vi "arydh -- get all readings.vi"(7 "nanocal config":T2={"Hs"={"out"=enum."D", "shunt R (Ohm)"=100000.0, "V"={"c"=enum."A V1", "l"=enum."Lock-in set L1"}, "\"I\""={"c"=enum."A V2", "l"=enum."Lock-in set L1"}}, "ofset heater"={"out"=enum."C", "\"I\""=enum."C V2", "shunt R (Ohm)"=10000.0}, "Ts"={"out"=enum."D", "shunt R (Ohm)"=100000.0, "V"={"c"=enum."D V1", "l"=enum."Lock-in set L1"}, "\"I\""={"c"=enum."D V2", "l"=enum."Lock-in set L1"}}, "Tr"={"out"=enum."B", "shunt R (Ohm)"=100000.0, "V"={"c"=enum."E V1", "l"=enum."Lock-in set L1"}, "\"I\""={"c"=enum."E V2", "l"=enum."Lock-in set L1"}}, "Hr"={"out"=enum."E", "shunt R (Ohm)"=100000.0, "V"={"c"=enum."B V1", "l"=enum."Lock-in set L1"}, "\"I\""={"c"=enum."B V2", "l"=enum."Lock-in set L1"}}, "differential"={"c"=enum."C V1", "l"=enum."Lock-in set L2"}} {"Hr"."shunt R (Ohm)" format="%#_6p"; "Tr"."shunt R (Ohm)" format="%#_6p"; "Ts"."shunt R (Ohm)" format="%#_6p"; "ofset heater"."shunt R (Ohm)" format="%#_6p"; "Hs"."shunt R (Ohm)" format="%#_6p"}, 11 "MCL object":T7) -> (2 "engine reading":T1={"Ts -- V (V)"=100000.0+0.0i, "Hr -- V (V)"=100000.0+0.0i, "Hs -- V (V)"=100000.0+0.0i, "Tr -- V (V)"=100000.0+0.0i, "Diff -- V (V)"=100000.0+0.0i, "offset (V)"=100000.0+0.0i, "Ts -- \"I\" (V)"=100000.0+0.0i, "Hs -- \"I\" (V)"=100000.0+0.0i, "Tr -- \"I\" (V)"=100000.0+0.0i, "Hr -- \"I\" (V)"=100000.0+0.0i, "freq (Hz)"=100000.0} {"freq (Hz)" format="%#_6p"; "Hr -- \"I\" (V)" format="%#_6p"; "Tr -- \"I\" (V)" format="%#_6p"; "Hs -- \"I\" (V)" format="%#_6p"; "Ts -- \"I\" (V)" format="%#_6p"; "offset (V)" format="%#_6p"; "Diff -- V (V)" format="%#_6p"; "Tr -- V (V)" format="%#_6p"; "Hs -- V (V)" format="%#_6p"; "Hr -- V (V)" format="%#_6p"; "Ts -- V (V)" format="%#_6p"})   [LabVIEW 2018]
uses:
  nanocal/Nanocalorimetry/data/MCL.lvlibp/MCL library/MCL_DataRef.ctl
  nanocal - config.ctl
  resistoricicle.ctl
  channelicicle.ctl
  nanocal/Nanocalorimetry/data/MCL.lvlibp/SynkTek FPGA/FPGA_SharedResources/FPGASharedResources_Readings_ReadingChannelTypedef.ctl
  nanocal/Nanocalorimetry/data/MCL.lvlibp/SynkTek FPGA/FPGA_SharedResources/FPGASharedResources_Lockin_Typedef.ctl
  engine reading icicle.ctl
  nanocal/Nanocalorimetry/data/MCL.lvlibp/SynkTek FPGA/FPGA_SharedResources/FPGASharedResources_FreqCtrl_FreqGenTypedef.ctl
  nanocal/Nanocalorimetry/data/MCL.lvlibp
  nanocal/Nanocalorimetry/data/MCL.lvlibp/SynkTek FPGA/FPGA_SharedResources/FPGA_SharedResources.lvlib
panel:
  # "Ts"
  # "Tr"
  # "Hs"
  # "Hr"
  # "offset heater"
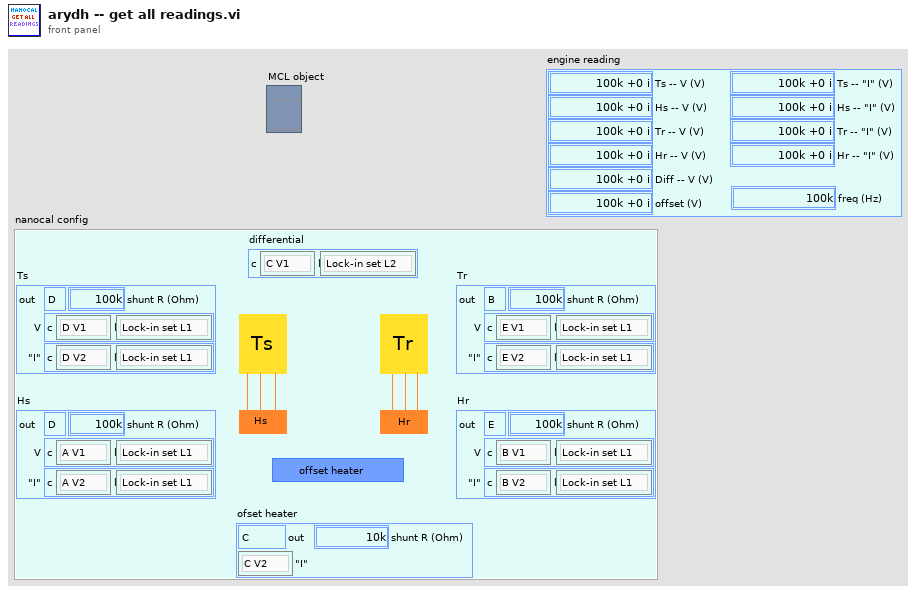
[diagram p1: front panel]
types:
  T1 = typedef "engine reading icicle.ctl" = cluster{"Ts -- V (V)":cdb, "Hr -- V (V)":cdb, "Hs -- V (V)":cdb, "Tr -- V (V)":cdb, "Diff -- V (V)":cdb, "offset (V)":cdb, "Ts -- \"I\" (V)":cdb, "Hs -- \"I\" (V)":cdb, "Tr -- \"I\" (V)":cdb, "Hr -- \"I\" (V)":cdb, "freq (Hz)":dbl}
  T2 = typedef "nanocal - config.ctl" = cluster{"Hs":T3, "ofset heater":cluster{"out":enum16{"A", "B", "C", "D", "E"}, "\"I\"":T5, "shunt R (Ohm)":dbl}, "Ts":T3, "Tr":T3, "Hr":T3, "differential":T4}
  T3 = typedef "resistoricicle.ctl" = cluster{"out":enum16{"A", "B", "C", "D", "E"}, "shunt R (Ohm)":dbl, "V":T4, "\"I\"":T4}
  T4 = typedef "channelicicle.ctl" = cluster{"c":T5, "l":T6}
  T5 = typedef "MCL.lvlibp/FPGA_SharedResources.lvlib/FPGASharedResources_Readings_ReadingChannelTypedef.ctl" = enum8{"A V1", "A V2", "B V1", "B V2", "C V1", "C V2", "D V1", "D V2", "E V1", "E V2", "A I", "B I", "C I", "D I", "E I", "Int."}
  T6 = typedef "MCL.lvlibp/FPGA_SharedResources.lvlib/FPGASharedResources_Lockin_Typedef.ctl" = enum8{"Lock-in set L1", "Lock-in set L2"}
  T7 = typedef "MCL.lvlibp/MCL_DataRef.ctl" = refnum<vi>
  T8 = typedef "MCL.lvlibp/FPGA_SharedResources.lvlib/FPGASharedResources_FreqCtrl_FreqGenTypedef.ctl" = enum8{"Frequency 1", "Frequency 2", "Frequency 3", "Frequency 4", "Frequency 5", "Frequency 6: PLL 1", "Frequency 7: PLL 2", "Frequency 8"}
  T9 = typedef "MCL.lvlibp/LIControl.lvlib/LIControl_FreqCtrl_typedef.ctl" = cluster{"Frequency (Hz)":dbl, "Ramp changes":bool, "Ramp time const. (s)":T10}
  T10 = typedef "MCL.lvlibp/LIControl.lvlib/LIControl_LockinTimeConstant_typedef.ctl" = dbl
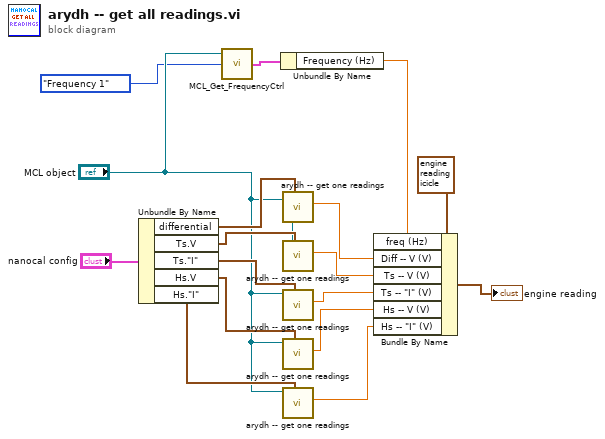
[diagram p0: block diagram]
diagram:
  n1 = Unbundle By Name("nanocal config") -> ("differential"=w15:T4, "Ts.V"=w13:T4, "Ts.\"I\""=w11:T4, "Hs.V"=w9:T4, "Hs.\"I\""=w8:T4)
  n2 = call "MCL_Get_FrequencyCtrl.vi"("Frequency generator"=FPGASharedResources_FreqCtrl_FreqGenTypedef."Frequency 1", "MCL object"="MCL object") -> ("FrequencyCtrl"=w2:T9)  [unwired: 1 in, 2 out]
  n3 = Unbundle By Name(w2) -> ("Frequency (Hz)"=w1:dbl)
  n4 = call "arydh -- get one readings.vi"("channelicicle"=w15, "MCL object"="MCL object") -> ("reading"=w14:cdb)  [unwired: 8 in, 1 out]
  n5 = call "arydh -- get one readings.vi"("channelicicle"=w13, "MCL object"="MCL object") -> ("reading"=w12:cdb)  [unwired: 8 in, 1 out]
  n6 = call "arydh -- get one readings.vi"("channelicicle"=w11, "MCL object"="MCL object") -> ("reading"=w10:cdb)  [unwired: 8 in, 1 out]
  n7 = call "arydh -- get one readings.vi"("channelicicle"=w9, "MCL object"="MCL object") -> ("reading"=w7:cdb)  [unwired: 8 in, 1 out]
  n8 = call "arydh -- get one readings.vi"("channelicicle"=w8, "MCL object"="MCL object") -> ("reading"=w6:cdb)  [unwired: 8 in, 1 out]
  n9 = Bundle By Name(cluster=T1 {"Ts -- V (V)"=100000.0+0.0i, "Hr -- V (V)"=100000.0+0.0i, "Hs -- V (V)"=100000.0+0.0i, "Tr -- V (V)"=100000.0+0.0i, "Diff -- V (V)"=100000.0+0.0i, "offset (V)"=100000.0+0.0i, "Ts -- \"I\" (V)"=100000.0+0.0i, "Hs -- \"I\" (V)"=100000.0+0.0i, "Tr -- \"I\" (V)"=100000.0+0.0i, "Hr -- \"I\" (V)"=100000.0+0.0i, "freq (Hz)"=100000.0} ("engine reading"), "freq (Hz)"=w1, "Diff -- V (V)"=w14, "Ts -- V (V)"=w12, "Ts -- \"I\" (V)"=w10, "Hs -- V (V)"=w7, "Hs -- \"I\" (V)"=w6) -> (→"engine reading":T1)
